vi "ImageNameConvertor.vi"(7 "time_stamp":bool=TRUE, 9 "postfix":string="tiff", 10 "filename":string="default", 11 "Path":path=path "E:/data/default") -> (2 "output":path=path "E:/data/default/default_27015021.tiff")   [LabVIEW 2014]
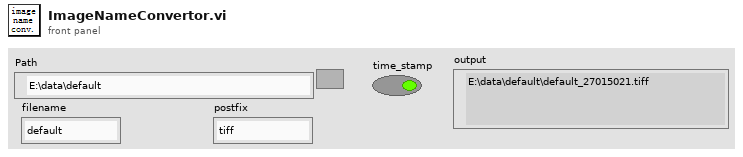
[diagram p1: front panel]
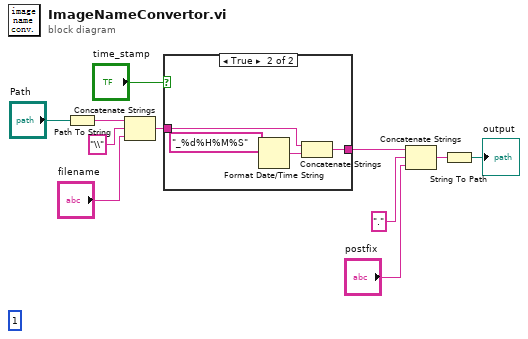
[diagram p0: block diagram]
diagram:
  (unwired) 1 ("compression (default)")
  n1 = Path To String(path="Path") -> (string=w4:string)
  n2 = Concatenate Strings(w4, "\\" ("string"), "filename") -> (w3:string)
  n3 = case shown="True" "time_stamp" {
    tunnel: w3 -> [w12 w14]
    tunnel: [w12 w13] -> w9
    frame False {
    }
    frame True {
      n4 = Format Date/Time String(time format string (%c)="_%d%H%M%S" ("时间格式字符串(%c)")) -> (date/time string=w16:string)  [unwired: 2 in]
      n5 = Concatenate Strings(w14, w16) -> (w13:string)
    }
  }
  n6 = Concatenate Strings(w9, "." ("string"), "postfix") -> (w7:string)
  n7 = String To Path(string=w7) -> (path=→"output":path)
